vi "ReplaceConstantNode.vi"(5 "Old Control Name":string, 7 "New Control Name":string, 8 "error in (no error)":errorcluster, 11 "VI Refnum In":refnum<vi>) -> (0 "error out":errorcluster, 3 "VI Refnum Out":refnum<vi>, 4 "Replaced":bool)   [LabVIEW 2024]
uses:
  <vilib>/Utility/traverseref.llb/TRef TravTarget.ctl
  <vilib>/Utility/traverseref.llb/VI Scripting - Traverse.lvlib
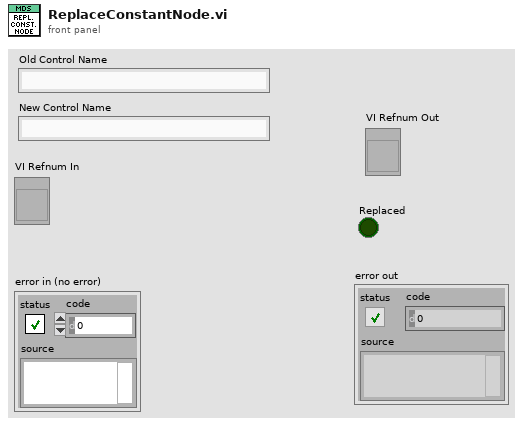
[diagram p1: front panel]
types:
  T1 = typedef "TRef TravTarget.ctl" = enum16{"FP", "BD", "Other"}
  T2 = enum32{"not a typedef", "typedef", "strict typedef", "class private data"}
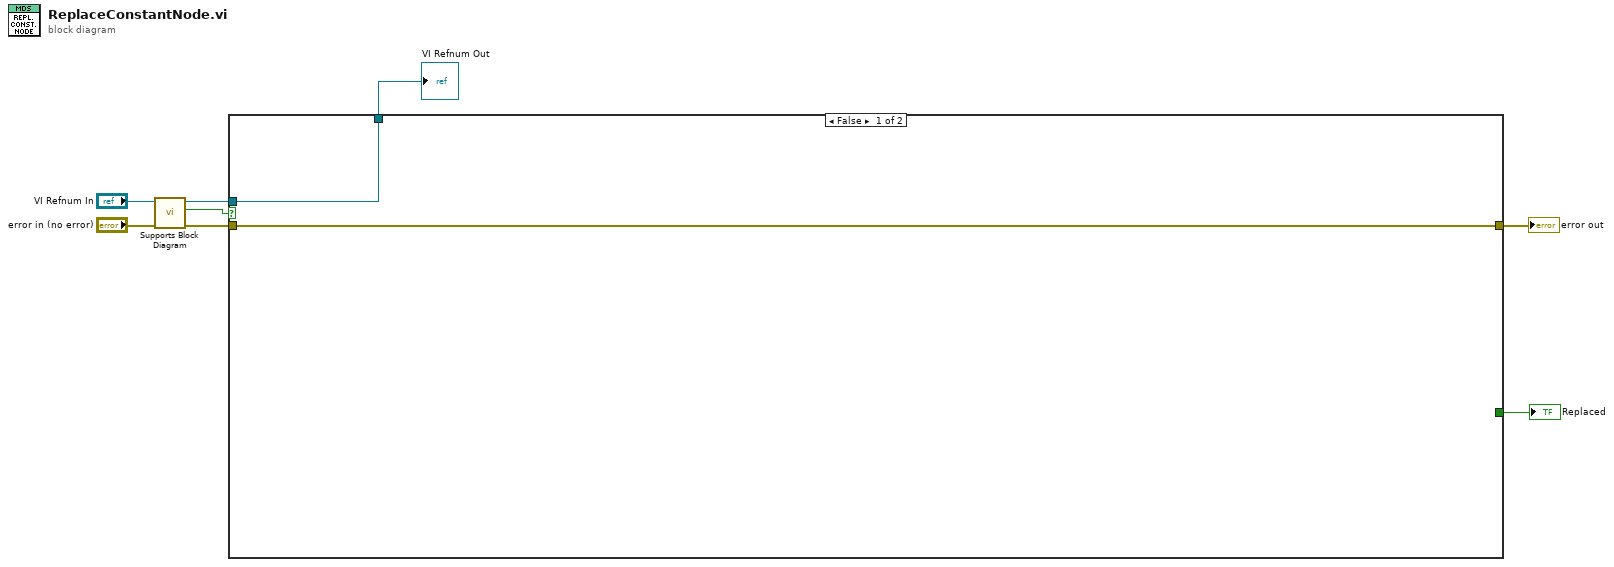
[diagram p0: block diagram]
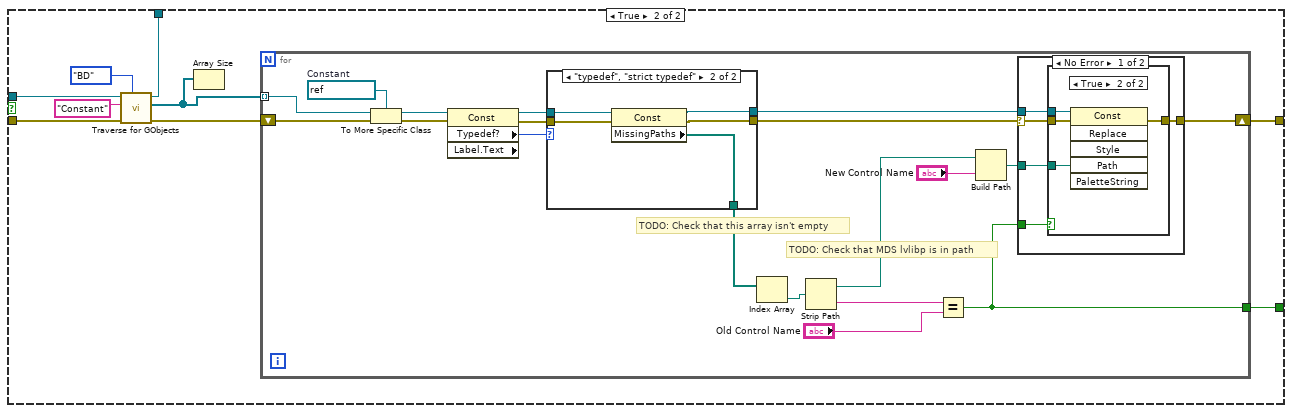
[diagram p2: hidden frame]
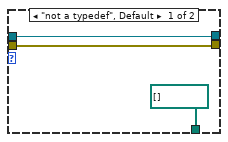
[diagram p3: hidden frame]
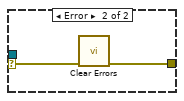
[diagram p5: hidden frame]
diagram:
  n1 = call "Supports Block Diagram.vi"("error in (no error)"="error in (no error)", "vi in"="VI Refnum In") -> ("error out"=w2:errorcluster, "has block diagram"=w1:bool, "vi out"=w3:refnum<vi>)  [unwired: 7 in]
  n2 = case shown="False" w1 {
    tunnel: [_ w16] -> w8
    tunnel: w2 -> [w9 w15]
    tunnel: w3 -> [w10 w14]
    tunnel: [w9 w12] -> w7
    tunnel: [w10 w11] -> w6
    frame False {
    }
    frame True {
      n3 = call <vilib>:"Traverse for GObjects.vi"("Traverse Target"=TRef_TravTarget."BD", "error in (no error)"=w15, "Class Name"="Constant", "VI Refnum"=w14) -> ("error out"=w19:errorcluster, "References"=w13:refnum<vi>[], "dup VI Refnum"=w11:refnum<vi>)  [unwired: 4 in, 1 out]
      n4 = Array Size(array=w13) -> ()  [unwired: 1 out]
      n5 = for {
        shift-right: [w33] -> w12
        shift-left: w19 -> [w37]
        tunnel: w13 -> [w38] mode=indexing
        tunnel: [w34] -> w16
        w29 = refnum<vi> refnum  # Constant
        # "TODO: Check that this array isn't empty"
        # "TODO: Check that MDS lvlibp is in path"
        n6 = To More Specific Class(target class=w29, reference=w38, error in=w37) -> (specific class reference=w28:refnum<vi>, error out=w27:errorcluster)
        n7 = property class="Const" props=["Typedef?", "Label", "Text"](reference=w28, error in=w27) -> (reference out=w24:refnum<vi>, error out=w26:errorcluster, "Typedef?"=w20:T2)  [unwired: 1 out]
        n8 = case shown="\"typedef\", \"strict typedef\"" w20 {
          tunnel: [path[] [] ("MissingPaths") w46] -> w22
          tunnel: w26 -> [w39 w45]
          tunnel: [w39 w44] -> w25
          tunnel: w24 -> [w40 w43]
          tunnel: [w40 w42] -> w23
          frame "not a typedef", Default {
          }
          frame "typedef", "strict typedef" {
            n9 = property class="Const"(reference=w43, error in=w45) -> (reference out=w42:refnum<vi>, error out=w44:errorcluster, "MissingPaths"=w46:path[])
          }
        }
        n10 = Index Array(array=w22) -> (element=w21:path)  [unwired: 1 in]
        n11 = Strip Path(path=w21) -> (stripped path=w30:path, name=w35:string)
        n12 = Equal?(x=w35, y="Old Control Name") -> (x = y?=w34:bool)
        n13 = Build Path(base path=w30, name or relative path="New Control Name") -> (appended path=w32:path)
        n14 = case shown="No Error" w25 {
          selector: w25 -> [w47 w58]
          tunnel: w32 -> [w51 _]
          tunnel: w34 -> [w50 _]
          tunnel: [w49 w57] -> w33
          tunnel: w23 -> [w48 _]
          frame No Error {
            n15 = case shown="True" w50 {
              tunnel: w51 -> [_ w56]
              tunnel: w47 -> [w52 w55]
              tunnel: [w52 w54] -> w49
              tunnel: w48 -> [_ w53]
              frame False {
              }
              frame True {
                n16 = invoke class="Const" method="Replace"(reference=w53, error in=w55, "Path"=w56) -> (error out=w54:errorcluster)  [unwired: 3 in, 5 out]
              }
            }
          }
          frame Error {
            n17 = call <vilib>:"Clear Errors.vi"("error in (no error)"=w58) -> ("error out"=w57:errorcluster)  [unwired: 5 in, 1 out]
          }
        }
      }
    }
  }
  "error out" <- w7
  "Replaced" <- w8
  "VI Refnum Out" <- w6
